vi "test-TimeInterpPose-Test2.vi"() -> (3 "All tests passed":bool)   [LabVIEW 2019]
uses:
  <vilib>/Rock Robotics/WPI/ThirdParty/JAS_Junk/TrajLib/TIME_INTERPOLATABLE_POSE.ctl
  <vilib>/Rock Robotics/WPI/ThirdParty/JAS_Junk/TrajLib/POSE2D.ctl
  <vilib>/Rock Robotics/WPI/ThirdParty/JAS_Junk/TrajLib/TRANSLATION2D.ctl
  <vilib>/Rock Robotics/WPI/ThirdParty/JAS_Junk/TrajLib/ROTATION2D.ctl
  <vilib>/Rock Robotics/WPI/ThirdParty/JAS_Junk/TrajLib/Rotation2d_CreateAngle.vi
  <vilib>/Rock Robotics/WPI/ThirdParty/JAS_Junk/TrajLib/Translation2d_Create.vi
  <vilib>/Rock Robotics/WPI/ThirdParty/JAS_Junk/TrajLib/TimeInterpPose2d_CleanUp.vi
  <vilib>/Rock Robotics/WPI/ThirdParty/JAS_Junk/TrajLib/MathUtil_InputModulus.vi
  <vilib>/gmath/interp.llb/Search Ordered Table.vi
  <vilib>/Rock Robotics/WPI/ThirdParty/JAS_Junk/TrajLib/Trajectory_Library.lvlib
panel:
  out "Add Error":bool
  out "Calc Pose":T1 {"ROTATION"."SIN" format="%13.4f"; "ROTATION"."COS" format="%13.4f"; "ROTATION"."VALUE" format="%13.4f"; "TRANSLATION"."Y" format="%14.3f"; "TRANSLATION"."X" format="%14.3f"}
  out "OutputPose":T1={"TRANSLATION"={"X"=0.0, "Y"=0.0}, "ROTATION"={"VALUE"=0.0, "COS"=1.0, "SIN"=0.0}} {"ROTATION"."SIN" format="%13.4f"; "ROTATION"."COS" format="%13.4f"; "ROTATION"."VALUE" format="%13.4f"; "TRANSLATION"."Y" format="%14.3f"; "TRANSLATION"."X" format="%14.3f"}
  out "Error 1":bool
  out "Error 2":bool
  out "TimeInterpPose":T4 {"Pose"."ROTATION"."SIN" format="%13.4f"; "Pose"."ROTATION"."COS" format="%13.4f"; "Pose"."ROTATION"."VALUE" format="%13.4f"; "Pose"."TRANSLATION"."Y" format="%14.3f"; "Pose"."TRANSLATION"."X" format="%14.3f"}
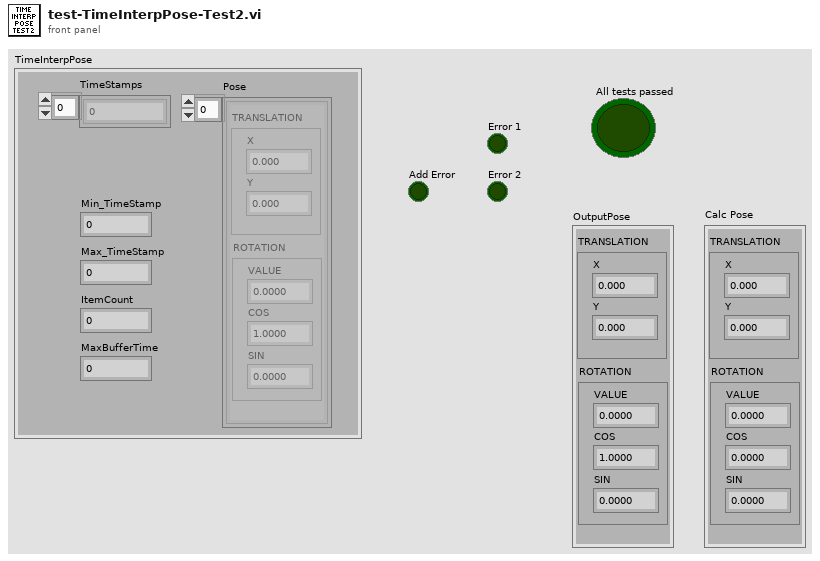
[diagram p1: front panel]
types:
  T1 = typedef "Trajectory_Library.lvlib/POSE2D.ctl" = cluster{"TRANSLATION":T2, "ROTATION":T3}
  T2 = typedef "Trajectory_Library.lvlib/TRANSLATION2D.ctl" = cluster{"X":dbl, "Y":dbl}
  T3 = typedef "Trajectory_Library.lvlib/ROTATION2D.ctl" = cluster{"VALUE":dbl, "COS":dbl, "SIN":dbl}
  T4 = typedef "Trajectory_Library.lvlib/TIME_INTERPOLATABLE_POSE.ctl" = cluster{"TimeStamps":dbl[], "Pose":T1[], "Min_TimeStamp":dbl, "Max_TimeStamp":dbl, "ItemCount":i32, "MaxBufferTime":dbl}
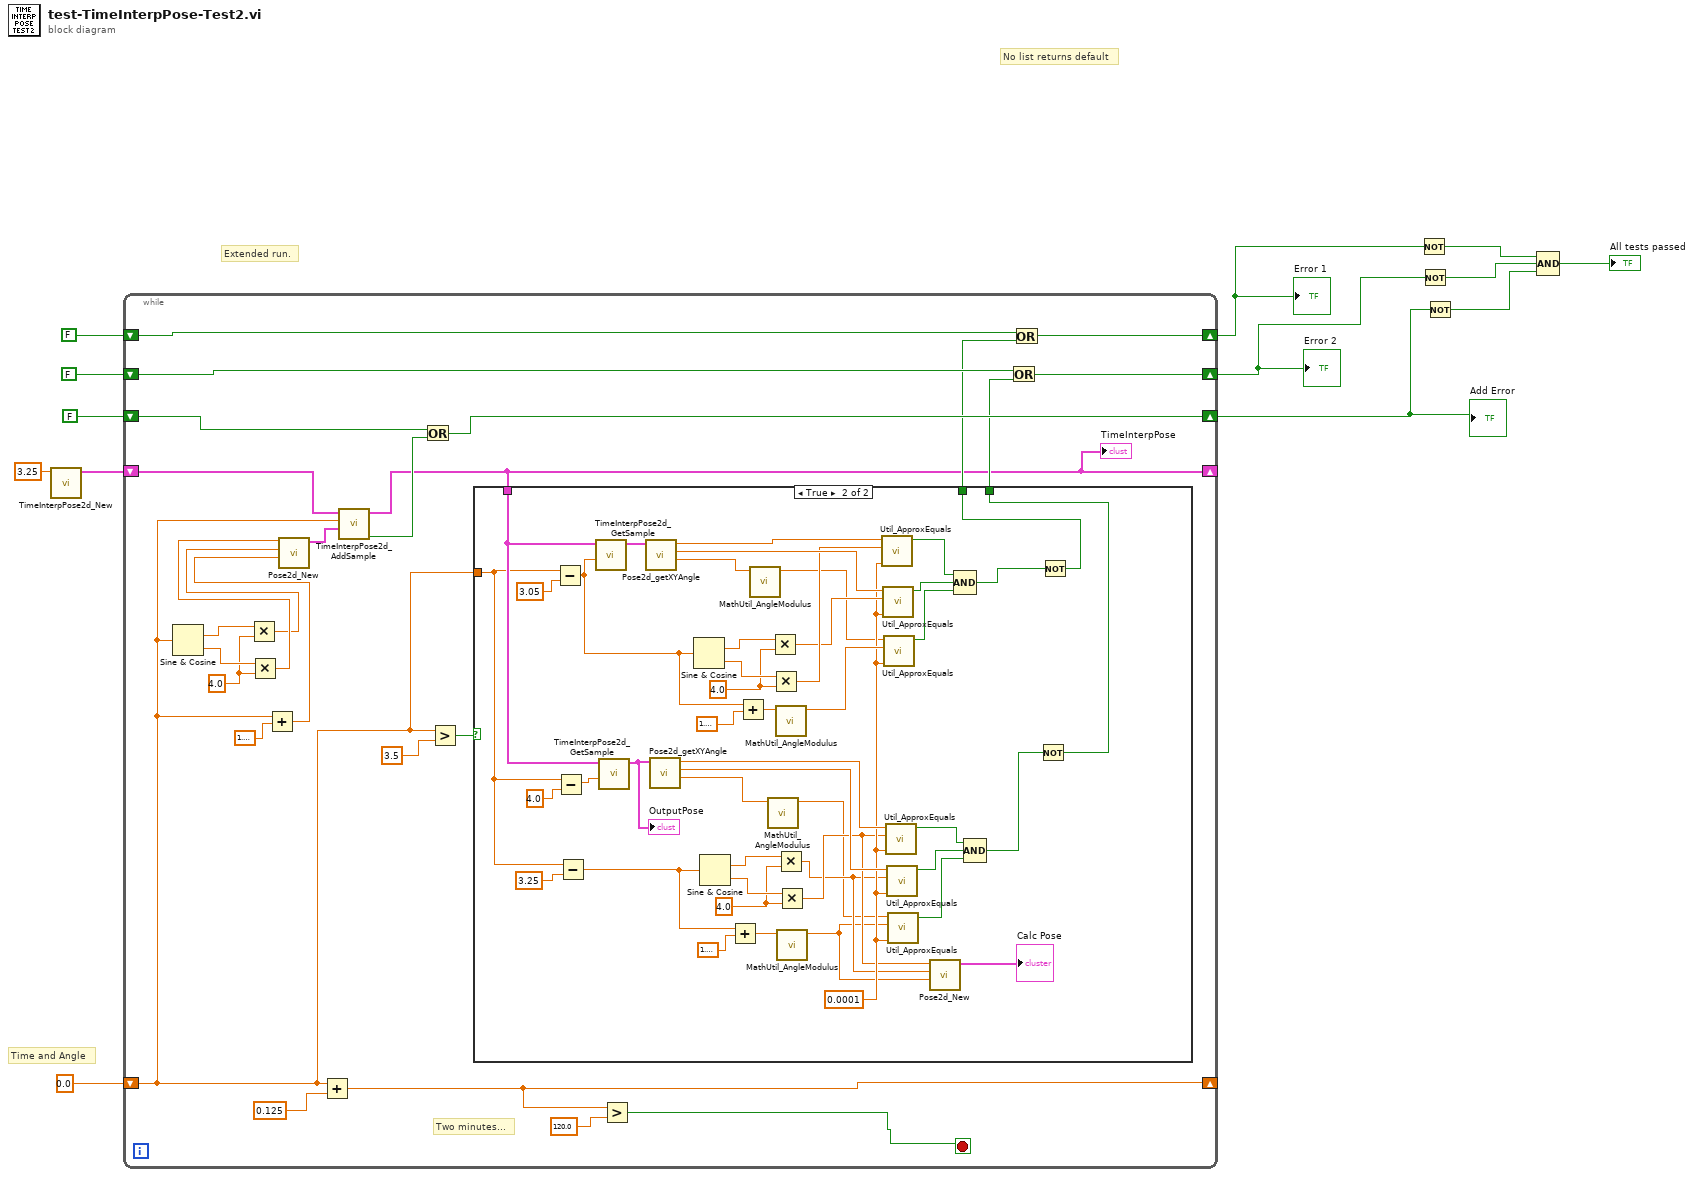
[diagram p0: block diagram]
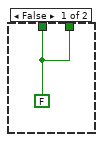
[diagram p2: hidden frame]
diagram:
  # "Extended run."
  # "Time and Angle"
  # "No list returns default"
  n1 = call <vilib>:"TimeInterpPose2d_New.vi"("MaxTime"=3.25) -> ("TimeInterpPose"=w11:T4)  [unwired: 10 in]
  n2 = while {
    shift-right: [w36] -> _
    shift-left: 0.0 -> [w22]
    shift-right: [w14] -> _
    shift-left: w11 -> [w34]
    shift-right: [w19] -> w7
    shift-left: FALSE -> [w25]
    shift-right: [w20] -> w5
    shift-left: FALSE -> [w17]
    shift-right: [w21] -> w6
    shift-left: FALSE -> [w18]
    stop <- w39 stop-if-true
    w31 = 4.0 ("y")
    # "Two minutes..."
    n3 = Sine & Cosine(0:w22) -> (1:w33:dbl, 2:w32:dbl)
    n4 = Multiply(x=w33, y=w31) -> (x*y=w29:dbl)
    n5 = Multiply(x=w32, y=w31) -> (x*y=w30:dbl)
    n6 = Add(x=w22, y=1.5707963267948966) -> (x+y=w27:dbl)
    n7 = call <vilib>:"Pose2d_New.vi"("Heading"=w27, "Y"=w29, "X"=w30) -> ("out POSe"=w35:T1)  [unwired: 8 in]
    n8 = Add(x=w22, y=0.125) -> (x+y=w36:dbl)
    n9 = call <vilib>:"TimeInterpPose2d_AddSample.vi"("Pose"=w35, "TimeStamp"=w22, "in TimeInterpPose"=w34) -> ("Error"=w26:bool, "out TimeInterpPose"=w14:T4)  [unwired: 7 in]
    "TimeInterpPose" <- w14
    n10 = Or(x=w25, y=w26) -> (x .or. y?=w19:bool)
    n11 = Greater?(x=w22, y=3.5) -> (0:w24:bool)
    n12 = case shown="True" w24 {
      tunnel: w14 -> [_ w86]
      tunnel: w22 -> [_ w72]
      tunnel: [w40 w43] -> w16
      tunnel: [w40 w41] -> w15
      frame False {
        w40 = FALSE
      }
      frame True {
        w60 = 0.0001 ("Tolerance")
        w74 = 4.0 ("y")
        w81 = 4.0 ("y")
        n13 = Subtract(x=w72, y=3.05) -> (x-y=w52:dbl)
        n14 = Subtract(x=w72, y=4.0) -> (x-y=w84:dbl)
        n15 = Subtract(x=w72, y=3.25) -> (x-y=w70:dbl)
        n16 = call <vilib>:"TimeInterpPose2d_GetSample.vi"("TimeStamp"=w52, "TimeInterpPose"=w86) -> ("OutputPose"=w79:T1)  [unwired: 9 in]
        n17 = call <vilib>:"TimeInterpPose2d_GetSample.vi"("TimeStamp"=w84, "TimeInterpPose"=w86) -> ("OutputPose"=w78:T1)  [unwired: 9 in]
        "OutputPose" <- w78
        n18 = call <vilib>:"Pose2d_getXYAngle.vi"("in POSE"=w79) -> ("Angle"=w45:dbl, "Y"=w68:dbl, "X"=w69:dbl)  [unwired: 8 in]
        n19 = call <vilib>:"Pose2d_getXYAngle.vi"("in POSE"=w78) -> ("Angle"=w47:dbl, "Y"=w61:dbl, "X"=w62:dbl)  [unwired: 8 in]
        n20 = Sine & Cosine(0:w52) -> (1:w83:dbl, 2:w82:dbl)
        n21 = Sine & Cosine(0:w70) -> (1:w76:dbl, 2:w75:dbl)
        n22 = Add(x=w70, y=1.5707963267948966) -> (x+y=w64:dbl)
        n23 = Add(x=w52, y=1.5707963267948966) -> (x+y=w65:dbl)
        n24 = call <vilib>:"MathUtil_AngleModulus.vi"("InputAngle"=w45) -> ("ModulsAngle"=w44:dbl)  [unwired: 10 in]
        n25 = call <vilib>:"MathUtil_AngleModulus.vi"("InputAngle"=w47) -> ("ModulsAngle"=w46:dbl)  [unwired: 10 in]
        n26 = Multiply(x=w83, y=w81) -> (x*y=w66:dbl)
        n27 = Multiply(x=w82, y=w81) -> (x*y=w67:dbl)
        n28 = call <vilib>:"MathUtil_AngleModulus.vi"("InputAngle"=w65) -> ("ModulsAngle"=w63:dbl)  [unwired: 10 in]
        n29 = Multiply(x=w76, y=w74) -> (x*y=w50:dbl)
        n30 = Multiply(x=w75, y=w74) -> (x*y=w51:dbl)
        n31 = call <vilib>:"MathUtil_AngleModulus.vi"("InputAngle"=w64) -> ("ModulsAngle"=w49:dbl)  [unwired: 10 in]
        n32 = call <vilib>:"Util_ApproxEquals.vi"("Tolerance"=w60, "Value 2"=w67, "Value 1"=w69) -> ("ApproxEquals"=w59:bool)  [unwired: 8 in]
        n33 = call <vilib>:"Util_ApproxEquals.vi"("Tolerance"=w60, "Value 2"=w66, "Value 1"=w68) -> ("ApproxEquals"=w58:bool)  [unwired: 8 in]
        n34 = call <vilib>:"Util_ApproxEquals.vi"("Tolerance"=w60, "Value 2"=w63, "Value 1"=w44) -> ("ApproxEquals"=w57:bool)  [unwired: 8 in]
        n35 = call <vilib>:"Util_ApproxEquals.vi"("Tolerance"=w60, "Value 2"=w51, "Value 1"=w62) -> ("ApproxEquals"=w54:bool)  [unwired: 8 in]
        n36 = call <vilib>:"Util_ApproxEquals.vi"("Tolerance"=w60, "Value 2"=w50, "Value 1"=w61) -> ("ApproxEquals"=w55:bool)  [unwired: 8 in]
        n37 = call <vilib>:"Util_ApproxEquals.vi"("Tolerance"=w60, "Value 2"=w49, "Value 1"=w46) -> ("ApproxEquals"=w56:bool)  [unwired: 8 in]
        n38 = call <vilib>:"Pose2d_New.vi"("Heading"=w49, "Y"=w50, "X"=w51) -> ("out POSe"=→"Calc Pose":T1)  [unwired: 8 in]
        n39 = Compound Arithmetic op=AND(w59, w58, w57) -> (w42:bool)
        n40 = Compound Arithmetic op=AND(w54, w55, w56) -> (w53:bool)
        n41 = Not(x=w53) -> (.not. x?=w41:bool)
        n42 = Not(x=w42) -> (.not. x?=w43:bool)
      }
    }
    n43 = Greater?(x=w36, y=120.0) -> (0:w39:bool)
    n44 = Or(x=w17, y=w15) -> (x .or. y?=w20:bool)
    n45 = Or(x=w18, y=w16) -> (x .or. y?=w21:bool)
  }
  "Add Error" <- w7
  "Error 1" <- w6
  "Error 2" <- w5
  n46 = Not(x=w6) -> (.not. x?=w4:bool)
  n47 = Not(x=w5) -> (.not. x?=w3:bool)
  n48 = Not(x=w7) -> (.not. x?=w2:bool)
  n49 = Compound Arithmetic op=AND(w4, w3, w2) -> (→"All tests passed":bool)
